vi "Prep Line Valve 0.vi"(8 "error in (no error)":errorcluster, 10 "Action (Read State)":enum16{"Read State", "Open", "Close"}(ring), 11 "cRIO-CO2 in":refnum<class "cRIO-CO2.lvclass">) -> (0 "error out":errorcluster, 2 "State":bool, 3 "cRIO-CO2 out":refnum<class "cRIO-CO2.lvclass">)   [LabVIEW 2015, in "cRIO-Carbondioxide.lvlib" / "cRIO-CO2.lvlib" / "cRIO-CO2.lvclass"]
uses:
  cRIO-CO2.lvclass
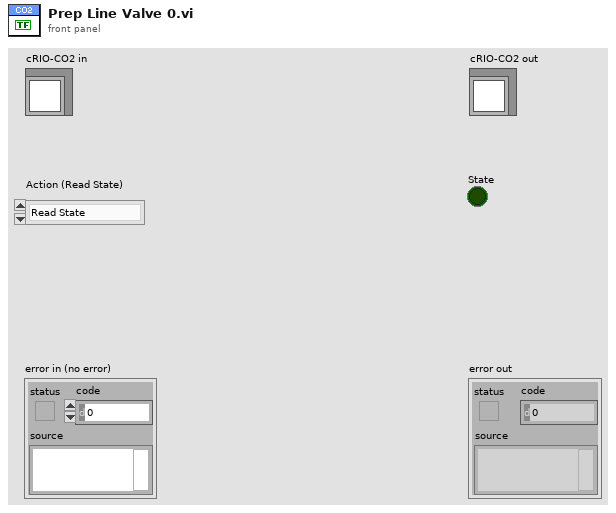
[diagram p1: front panel]
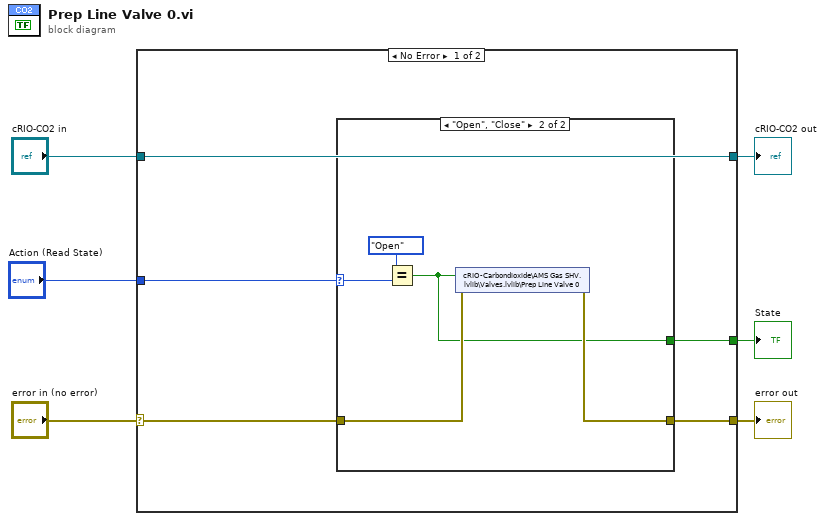
[diagram p0: block diagram]
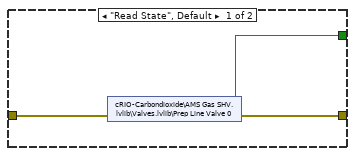
[diagram p2: hidden frame]
diagram:
  n1 = case shown="No Error" "error in (no error)" {
    selector: "error in (no error)" -> [w8 w21]
    tunnel: [w10 w21] -> w5
    tunnel: [w11 w20] -> w3
    tunnel: "cRIO-CO2 in" -> [w11 w20]
    tunnel: "Action (Read State)" -> [w9 _]
    tunnel: [w7 _] -> w1
    frame No Error {
      n2 = case shown="\"Open\", \"Close\"" w9 {
        selector: w9 -> [_ w17]
        tunnel: w8 -> [w14 w19]
        tunnel: [w13 w18] -> w10
        tunnel: [w12 w15] -> w7
        frame "Read State", Default {
          n3 = shared-variable "cRIO-Carbondioxide\\AMS Gas SHV.lvlib\\Valves.lvlib\\Prep Line Valve 0"(error in=w14) -> (w12:bool, error out=w13:errorcluster)
        }
        frame "Open", "Close" {
          n4 = Equal?(x=enum16{"Read State", "Open", "Close"}."Open", y=w17) -> (x = y?=w15:bool)
          n5 = shared-variable "cRIO-Carbondioxide\\AMS Gas SHV.lvlib\\Valves.lvlib\\Prep Line Valve 0"(w15, error in=w19) -> (error out=w18:errorcluster)
        }
      }
    }
    frame Error {
    }
  }
  "error out" <- w5
  "cRIO-CO2 out" <- w3
  "State" <- w1
